vi "Create AXI4-Stream Writer FXP32x1 v1 FPGA.vi"(9 "tdata":refnum<k21>, 10 "tvalid":refnum<k21>, 11 "niInstr AXI4-Stream Writer FXP32x1 v1 FPGA in":refnum<class "niInstr AXI4-Stream Writer FXP32x1 v1 FPGA.lvclass">) -> (3 "niInstr AXI4-Stream Writer FXP32x1 v1 FPGA out":refnum<class "niInstr AXI4-Stream Writer FXP32x1 v1 FPGA.lvclass">)   [LabVIEW 2015, in "niInstr AXI4-Stream Writer FXP32x1 v1 FPGA.lvclass"]
uses:
  <instrlib>/_niInstr/CLIP Adapters/v1/FPGA/AXI4-Stream/Writer FXP32x1/niInstr AXI4-Stream Writer FXP32x1 v1 FPGA.lvclass
  <instrlib>/_niInstr/CLIP Adapters/v1/FPGA/AXI4-Stream/Writer FXP32x1/niInstr AXI4-Stream Writer FXP32x1 v1 FPGA.lvclass/niInstr AXI4-Stream Writer FXP32x1 v1 FPGA.ctl
  <instrlib>/_niInstr/CLIP Adapters/v1/FPGA/AXI4-Stream/Writer/niInstr AXI4-Stream Writer v1 FPGA.lvclass
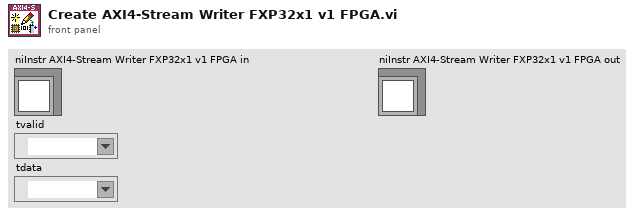
[diagram p1: front panel]
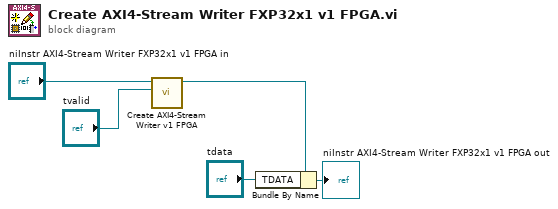
[diagram p0: block diagram]
diagram:
  n1 = call <instrlib>:"Create AXI4-Stream Writer v1 FPGA.vi"("tvalid"="tvalid", "niInstr AXI4-Stream Writer v1 FPGA in"="niInstr AXI4-Stream Writer FXP32x1 v1 FPGA in") -> ("niInstr AXI4-Stream Writer v1 FPGA out"=w3:refnum<class "niInstr AXI4-Stream Writer FXP32x1 v1 FPGA.lvclass">)  [unwired: 9 in]
  n2 = Bundle By Name(cluster=w3, "TDATA"="tdata") -> (→"niInstr AXI4-Stream Writer FXP32x1 v1 FPGA out":refnum<class "niInstr AXI4-Stream Writer FXP32x1 v1 FPGA.lvclass">)
